vi "InsideBoundaries.vi"(9 "Mouse Move Coords":T2, 11 "AntsRect":T1) -> (2 "Inside?":bool)   [LabVIEW 2021, in "Ants.lvclass"]
uses:
  Ants.lvclass
  <vilib>/Utility/miscctls.llb/LVPoint32TypeDef.ctl
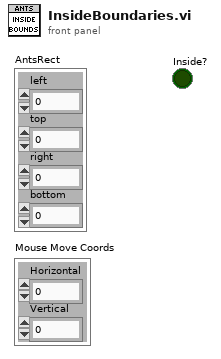
[diagram p1: front panel]
types:
  T1 = cluster{"left":i16, "top":i16, "right":i16, "bottom":i16}
  T2 = typedef "LVPoint32TypeDef.ctl" = cluster{"Horizontal":i32, "Vertical":i32}
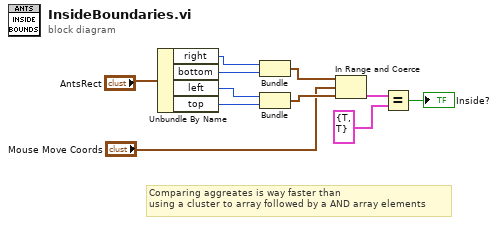
[diagram p0: block diagram]
diagram:
  # "Comparing aggreates is way faster than\nusing a cluster to array followed by a AND array elements"
  n1 = Unbundle By Name("AntsRect") -> ("right"=w7:i16, "bottom"=w8:i16, "left"=w9:i16, "top"=w10:i16)
  n2 = Bundle("right"=w7, "bottom"=w8) -> (w6:cluster{"right":i16, "bottom":i16})  [unwired: 1 out]
  n3 = Bundle("left"=w9, "top"=w10) -> (w5:cluster{"left":i16, "top":i16})  [unwired: 1 out]
  n4 = In Range and Coerce(upper limit=w6, x="Mouse Move Coords", lower limit=w5) -> (In Range?=w3:cluster{"Horizontal":bool, "Vertical":bool})  [unwired: 1 out]
  n5 = Equal?(x=w3, y=cluster{"Horizontal":bool, "Vertical":bool} {"Horizontal"=TRUE, "Vertical"=TRUE} ("In Range?")) -> (x = y?=→"Inside?":bool)
